vi "LED_blink5.vi"(8 "Error In":errorcluster, 9 "LEDs":bool[](array[boolean])=[FALSE, FALSE, FALSE, FALSE], 10 "Amount":u32=5, 11 "Time (ms)":u32=2500) -> (0 "Error Out":errorcluster)   [LabVIEW 2013]
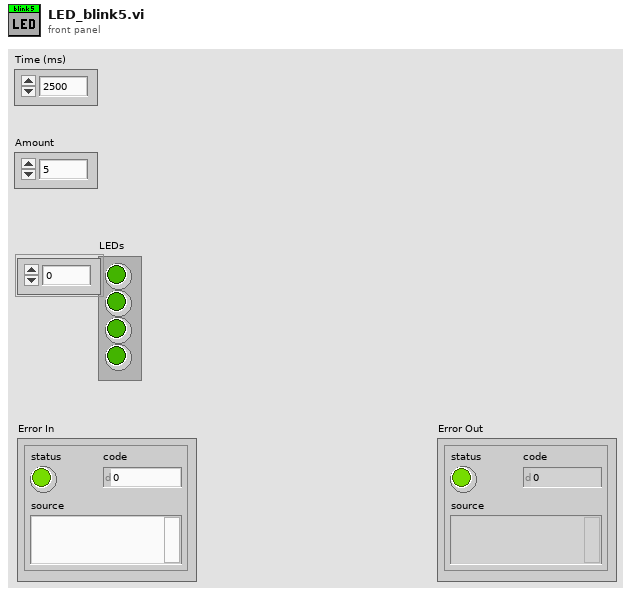
[diagram p1: front panel]
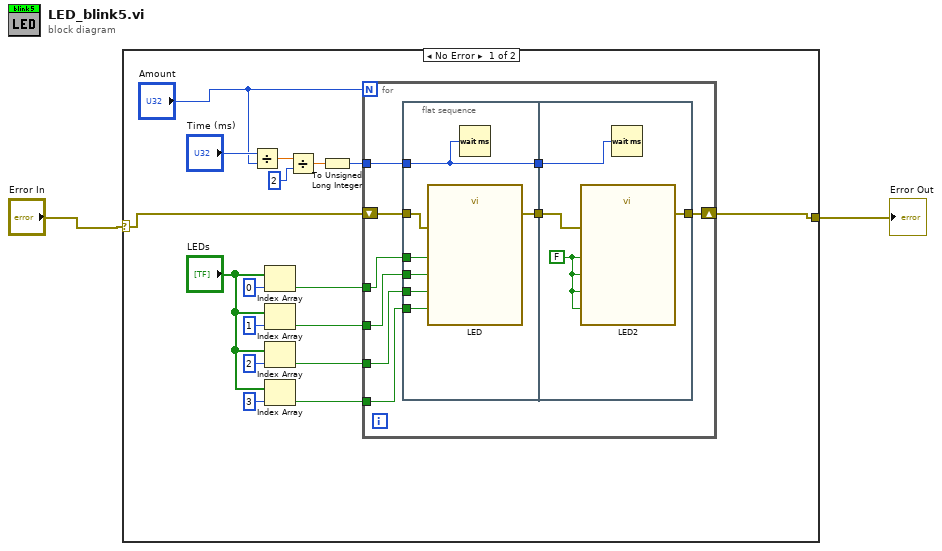
[diagram p0: block diagram]
diagram:
  n1 = case shown="No Error" "Error In" {
    selector: "Error In" -> [w4 w40]
    tunnel: [w19 w40] -> w2
    frame No Error {
      n2 = Divide(x="Time (ms)", y="Amount") -> (x/y=w18:dbl)
      n3 = Index Array(array="LEDs", index=0) -> (element=w8:bool)
      n4 = Index Array(array="LEDs", index=1) -> (element=w7:bool)
      n5 = Index Array(array="LEDs", index=2) -> (element=w6:bool)
      n6 = Index Array(array="LEDs", index=3) -> (element=w5:bool)
      n7 = Divide(x=w18, y=u8 2) -> (x/y=w15:dbl)
      n8 = To Unsigned Long Integer(number=w15) -> (unsigned 32bit integer=w14:u32)
      n9 = for {
        N: "Amount" -> [_]
        tunnel: w8 -> [w25]
        tunnel: w7 -> [w24]
        tunnel: w6 -> [w23]
        tunnel: w5 -> [w22]
        shift-right: [w27] -> w19
        shift-left: w4 -> [w28]
        tunnel: w14 -> [w20]
        n10 = flat-sequence {
          tunnel: w28 -> [w35]
          tunnel: [w34] -> w26
          tunnel: w25 -> [w33]
          tunnel: w24 -> [w32]
          tunnel: w23 -> [w31]
          tunnel: w22 -> [w30]
          tunnel: [w29] -> w21
          tunnel: w20 -> [w29]
          tunnel: [w39] -> w27
          tunnel: w26 -> [w38]
          tunnel: w21 -> [w36]
          frame #0 {
            n11 = call "LED"("LED0"=w33, "LED1"=w32, "LED2"=w31, "LED3"=w30, "error in (no error)"=w35) -> ("error out"=w34:errorcluster)  [unwired: 22 in]
            n12 = Wait (ms)(milliseconds to wait=w29) -> ()  [unwired: 1 out]
          }
          frame #1 {
            w37 = FALSE ("LED0")
            n13 = call "LED2"("LED0"=w37, "LED1"=w37, "LED2"=w37, "LED3"=w37, "error in (no error)"=w38) -> ("error out"=w39:errorcluster)  [unwired: 22 in]
            n14 = Wait (ms)(milliseconds to wait=w36) -> ()  [unwired: 1 out]
          }
        }
      }
    }
    frame Error {
    }
  }
  "Error Out" <- w2
